vi "Build ADU_RTU.vi"(8 "error in (no error)":errorcluster, 9 "Baud Rate (bps)":u32=19200, 10 "Slave Address":u8) -> (0 "error out":errorcluster, 3 "MB_ADU_RTU out":refnum<class "MB_ADU_RTU.lvclass">)   [LabVIEW 2023, in "Jiaxin_Stepper_Controller.lvlib" / "MB Master.lvlib" / "MB_ADU_RTU.lvclass"]
doc: "Builds an ADU for Modbus RTU mode"
uses:
  MB_ADU_RTU.lvclass
  C:/Users/quantum/Documents/LVDAQ/ConcreteClasses/ConcreteInstrumentClasses/Jiaxin_Stepper_Controller/Plasmionique/MB Master/MB_ADU/MB_ADU.lvclass
  MB_ADU/MB_ADU.lvclass/MB_ADU.ctl
  MB_ADU_RTU.lvclass/MB_ADU_RTU.ctl
  MB_ADU/MB_ADU.lvclass
panel:
  in  "MB_ADU_RTU in":refnum<class "MB_ADU_RTU.lvclass">
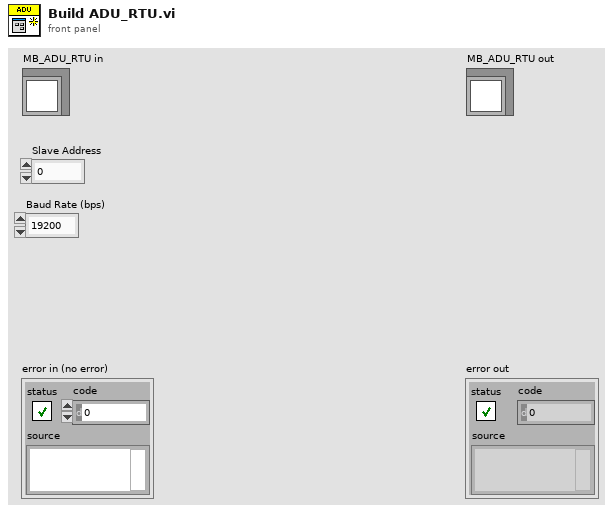
[diagram p1: front panel]
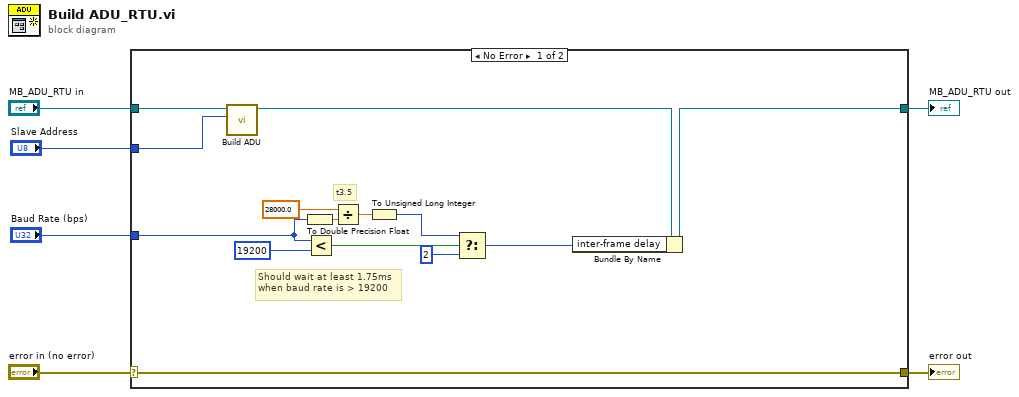
[diagram p0: block diagram]
diagram:
  n1 = case shown="No Error" "error in (no error)" {
    selector: "error in (no error)" -> [w20 w22]
    tunnel: [w20 w22] -> w5
    tunnel: [w16 w21] -> w3
    tunnel: "MB_ADU_RTU in" -> [w18 w21]
    tunnel: "Slave Address" -> [w19 _]
    tunnel: "Baud Rate (bps)" -> [w8 _]
    frame No Error {
      # "Should wait at least 1.75ms\nwhen baud rate is > 19200"
      # "t3.5"
      n2 = call "Build ADU.vi"("Slave ID"=w19, "MB_ADU in"=w18) -> ("MB_ADU out"=w17:refnum<class "MB_ADU_RTU.lvclass">)  [unwired: 8 in, 1 out]
      n3 = To Double Precision Float(number=w8) -> (double precision float=w10:dbl)
      n4 = Less?(x=w8, y=u32 19200) -> (x < y?=w14:bool)
      n5 = Divide(x=28000.0 ("y"), y=w10) -> (x/y=w12:dbl)
      n6 = To Unsigned Long Integer(number=w12) -> (unsigned 32bit integer=w9:u32)
      n7 = Select(t=w9, s=w14, f=u32 2 ("inter-frame delay")) -> (s? t:f=w7:u32)
      n8 = Bundle By Name(cluster=w17, "inter-frame delay"=w7) -> (w16:refnum<class "MB_ADU_RTU.lvclass">)
    }
    frame Error {
    }
  }
  "error out" <- w5
  "MB_ADU_RTU out" <- w3
